vi "Client Configure Read.vi"(7 "force configure? (F)":bool, 8 "error in":errorcluster, 11 "connection ID in":T1) -> (0 "error out":errorcluster, 1 "reconfigured?":bool, 3 "connection ID out":T1, 4 "read group name":string)   [LabVIEW 2010, in "NI_CCC.lvlib"]
uses:
  NI_CCC.lvlib
  Connection ID.ctl
  <vilib>/NI/STM/TCP/TCP Connection Info.ctl
  <vilib>/NI/STM/SubVIs/MetaDataElement.ctl
  Tag Configuration.ctl
  <vilib>/NI/Current Value Table/Type Defs/Data Types.ctl
  Tag Direction.ctl
  FG Client Configurations Action.ctl
  <vilib>/NI/STM/TCP/TCP Write Options.ctl
  <vilib>/NI/Current Value Table/Get Index and Type.vi
  <vilib>/NI/Current Value Table/Group Tags.vi
  <vilib>/NI/Current Value Table/FGVs/Tag Memory.vi
  <vilib>/Utility/error.llb/Error Cluster From Error Code.vi
  <vilib>/NI/Current Value Table/FGVs/Group Memory.vi
  <vilib>/NI/Current Value Table/Form Single Group.vi
  <vilib>/NI/STM/TCP/Read Message (TCP).vi
  <vilib>/NI/STM/NI STM.lvlib
  <vilib>/NI/Current Value Table/Current Value Table.lvlib
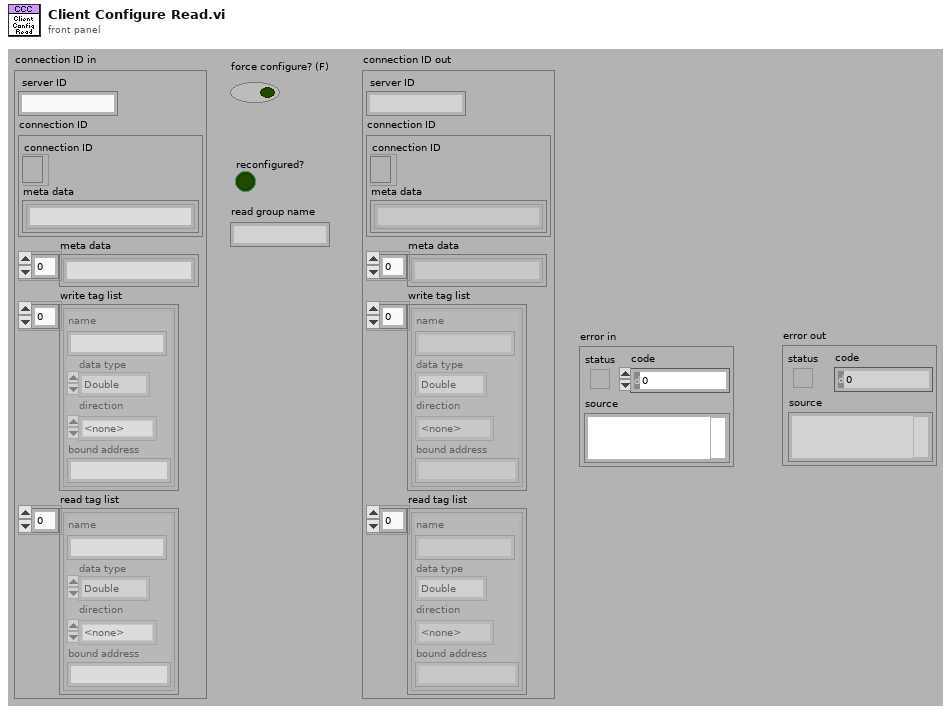
[diagram p1: front panel]
types:
  T1 = typedef "NI_CCC.lvlib/Connection ID.ctl" = cluster{"server ID":string, "connection ID":T2, "meta data":T3[], "write tag list":T4[], "read tag list":T4[]}
  T2 = typedef "NI STM.lvlib/TCP Connection Info.ctl" = cluster{"connection ID":refnum<k5>, "meta data":T3[]}
  T3 = typedef "NI STM.lvlib/MetaDataElement.ctl" = string
  T4 = typedef "NI_CCC.lvlib/Tag Configuration.ctl" = cluster{"name":string, "data type":T5, "direction":T6, "bound address":string}
  T5 = typedef "Current Value Table.lvlib/Data Types.ctl" = enum16{"Double", "Single", "I64", "I32", "I16", "I8", "U64", "U32", "U16", "U8", "String", "Boolean", "Array of U8", "Array of U16", "Array of U32", "Array of U64", "Array of I64", "Array of I32", "Array of I16", "Array of I8", "Array of Double", "Array of Single", "Array of Boolean", "Array of String"}
  T6 = typedef "NI_CCC.lvlib/Tag Direction.ctl" = enum32{"<none>", "Read", "Write"}
  T7 = typedef "NI_CCC.lvlib/FG Client Configurations Action.ctl" = enum16{"Check Read Config", "Check Write Config", "Mark Read Config", "Mark Write Config"}
  T8 = typedef "NI STM.lvlib/TCP Write Options.ctl" = cluster{"ignore timeout error":bool, "timeout ms (1000)":i32}
  T9 = typedef "NI_CCC.lvlib/Configure Read_Write Message.ctl" = cluster{"items":T10[]}
  T10 = typedef "NI_CCC.lvlib/Type_Tag.ctl" = cluster{"Data Type":T5, "tag":string}
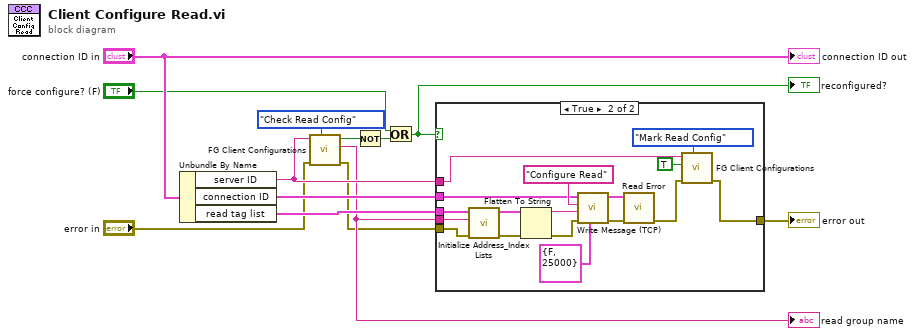
[diagram p0: block diagram]
diagram:
  n1 = Unbundle By Name("connection ID in") -> ("server ID"=w11:string, "connection ID"=w12:T2, "read tag list"=w13:T4[])
  n2 = call "FG Client Configurations.vi"("action"=FG_Client_Configurations_Action."Check Read Config", "error in"="error in", "server ID"=w11) -> ("error out"=w6:errorcluster, "group name"=w10:string, "configured?"=w7:bool)  [unwired: 6 in]
  "read group name" <- w10
  n3 = Not(x=w7) -> (.not. x?=w8:bool)
  n4 = Or(x="force configure? (F)", y=w8) -> (x .or. y?=w9:bool)
  "reconfigured?" <- w9
  n5 = case shown="True" w9 {
    tunnel: w13 -> [_ w24]
    tunnel: w6 -> [w14 w23]
    tunnel: [w14 w17] -> w1
    tunnel: w12 -> [_ w28]
    tunnel: w10 -> [_ w20]
    tunnel: w11 -> [_ w16]
    frame False {
    }
    frame True {
      n6 = call "Initialize Address_Index Lists.vi"("error in"=w23, "group name"=w20, "tag list"=w24) -> ("error out"=w22:errorcluster, "config server message"=w21:T9)  [unwired: 7 in]
      n7 = Flatten To String(anything=w21, error in (no error)=w22) -> (data string=w30:string, error out=w29:errorcluster)  [unwired: 3 out]
      n8 = call <vilib>:"Write Message (TCP).vi"("options"=T8 {"ignore timeout error"=FALSE, "timeout ms (1000)"=25000} ("Options"), "error in"=w29, "data"=w30, "name"="Configure Read" ("Name"), "connection info in"=w28) -> ("error out"=w26:errorcluster, "connection info out"=w27:T2)  [unwired: 5 in]
      n9 = call "Read Error.vi"("error in"=w26, "connection ID in"=w27) -> ("error out"=w18:errorcluster)  [unwired: 1 in, 8 out]
      n10 = call "FG Client Configurations.vi"("action"=FG_Client_Configurations_Action."Mark Read Config", "error in"=w18, "mark configured? (T)"=TRUE, "server ID"=w16) -> ("error out"=w17:errorcluster)  [unwired: 5 in, 2 out]
    }
  }
  "error out" <- w1
  "connection ID out" <- "connection ID in"
